vi "CSM - Request CSM to Broadcast Status Change.vi"(4 "Immediately? (F)":bool, 6 "Broadcast? (T)":bool=TRUE, 7 "Module Name":string, 8 "Error In (No Error)":errorcluster, 9 "Priority (\"Status\")":T1=enum."Status", 10 "Arguments (\"\")":string, 11 "Status":string="DoA") -> (0 "error out":errorcluster)   [LabVIEW 2017, in "Communicable State Machine.lvlib"]
doc: "Requests the CSM to send a broadcast. This VI is primarily used in CSM Multi-Loop Mode for other modules to request the CSM to issue a broadcast notifying other modules of a status change.\n\n> [!WARNING] As long as you know the module name, you can use this VI outside the CSM module to spoof a broadcast message from this module. However, this is not recommended because such logic makes the overall logic chaotic and increases debugging difficulty. Therefore, it is only recommended to use this VI in CSM Multi-Loop Mode.\n\n<b>Reference Example</b>: `4. Advance Examples\\5. Multi-Loop Module Example\\TCP Server Module(Multi-Loop Support).vi`.\n\n\n> [!NOTE] <b>CSM Multi-Loop Mode</b>\n>\n> In some scenarios, it is suitable to use multiple loops to constitute the same CSM module. For example:\n> - Retrofitting existing functional code into a CSM module. For example, TCP connection loops or DAQmx data acquisition loops. To ensure the clarity of the original logic, you can wrap the existing code in a While loop and append a CSM communication loop to implement the retrofitted functionality.\n> - In cases with high real-time requirements where a Timed Loop is needed, the CSM loop is required as a communication interface, while the Timed Loop serves as the functional loop implementation scheme.\n> - In cases where UI operations are very complex, it is recommended to separate UI operations from the CSM communication loop. The UI operation loop handles UI actions and generates inter-module messages, while the CSM loop serves as the actual functional loop.\n>\n> The Multi-Loop Support Mode API is used in such scenarios to pass internal messages between internal loops of a module or to provide CSM interface functionality for non-CSM loops.\n\n\n-- <b>Controls</b> --\n- <b>Module Name</b>: The CSM sending the status.\n- <b>Status</b>: Status to be broadcast.\n- <b>Arguments (\"\")</b>: Status arguments to be broadcast.\n- <b>Broadcast? (T)</b>: Switch input to control whether to broadcast.\n- <b>Immediately? (F)</b>: Immediate execution option. Sending immediately causes this message to be processed instantly in the CSM loop, rather than waiting for existing messages in the CSM loop to finish execution."
uses:
  Communicable State Machine.lvlib
  CSM - Broadcast Message Type.ctl
  _Support/CSMQ/_CSMOFGVOPER.ctl
  _Support/Typedef/_Cross CSM State Data.ctl
  _Support/Typedef/_CSM_MSG_TYPE.ctl
  _Support/Typedef/_Cross CSM State Response.ctl
  _Support/Typedef/_CSM_Response Source Message.ctl
  _Shared/CSM Shared.lvlib
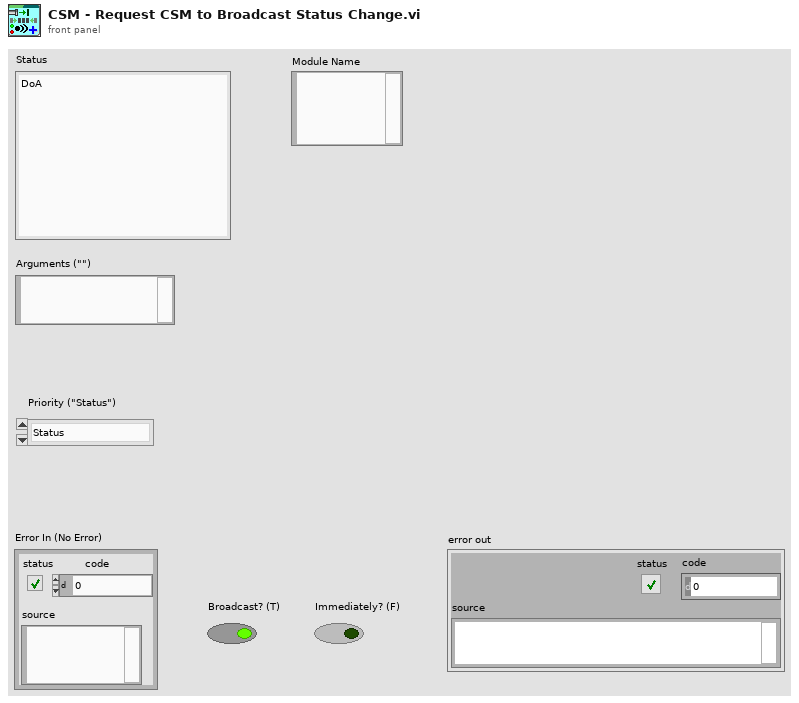
[diagram p1: front panel]
types:
  T1 = typedef "Communicable State Machine.lvlib/CSM - Broadcast Message Type.ctl" = enum16{"<Null>", "Status", "Interrupt"}
  T2 = typedef "Communicable State Machine.lvlib/_CSM_MSG_TYPE.ctl" = enum16{"Sync Message(-@)", "Async Message(->)", "Async without Response(->|)", "Async Response", "Broadcast(-><all>)", "Broadcast(-><status>)", "Broadcast(-><interrupt>)", "Append to JKISM States", "Append to JKISM States(High Priority)", "Broadcast(-><state>)"}
  T3 = typedef "Communicable State Machine.lvlib/_Cross CSM State Data.ctl" = cluster{"Msg Type":T2, "state":string, "args":string, "source":string, "RespQ":refnum<queue>, "Response For Message":T4, "Target":string}
  T4 = typedef "Communicable State Machine.lvlib/_CSM_Response Source Message.ctl" = cluster{"‘State":string, "’Arguments":string, "’Error":errorcluster}
  T5 = typedef "Communicable State Machine.lvlib/_CSMOFGVOPER.ctl" = enum16{"Create If not Exist", "Get By Name", "List", "Check If Name Exists", "Release", "Module Status", "Create Status Event Handler", "Destroy Status Event Handler", "Clear Invalid Objs"}
  T6 = typedef "Communicable State Machine.lvlib/_CSMObj.ctl" = cluster{"info":T7, "Refs":T9}
  T7 = typedef "Communicable State Machine.lvlib/_CSMObj-Info.ctl" = cluster{"Module Name":string, "Requested Name":string, "Group Name":string, "Mode":T8, "Allowed Messages":string[]}
  T8 = typedef "Communicable State Machine.lvlib/_CSM_MODE.ctl" = enum16{"Not Exist", "Stand Alone", "CSM", "Worker", "Worker Agent", "Chain Node", "Chain"}
  T9 = typedef "Communicable State Machine.lvlib/_CSMObj-Refs.ctl" = cluster{"WatchDogQ":refnum<queue>, "CSMDataDVR":refnum<data-value>, "Queue":T10, "GroupDataDVR":refnum<data-value>, "TagMap":refnum<data-value>, "ExitEvent":refnum<user-event>, "NewStateEvent":refnum<user-event>, "StatusEvent":refnum<user-event>, "InterruptEvent":refnum<user-event>}
  T10 = typedef "Communicable State Machine.lvlib/Priority Queue.ctl" = cluster{"HPriorityQ":refnum<queue>, "LowPriorityQ":refnum<queue>}
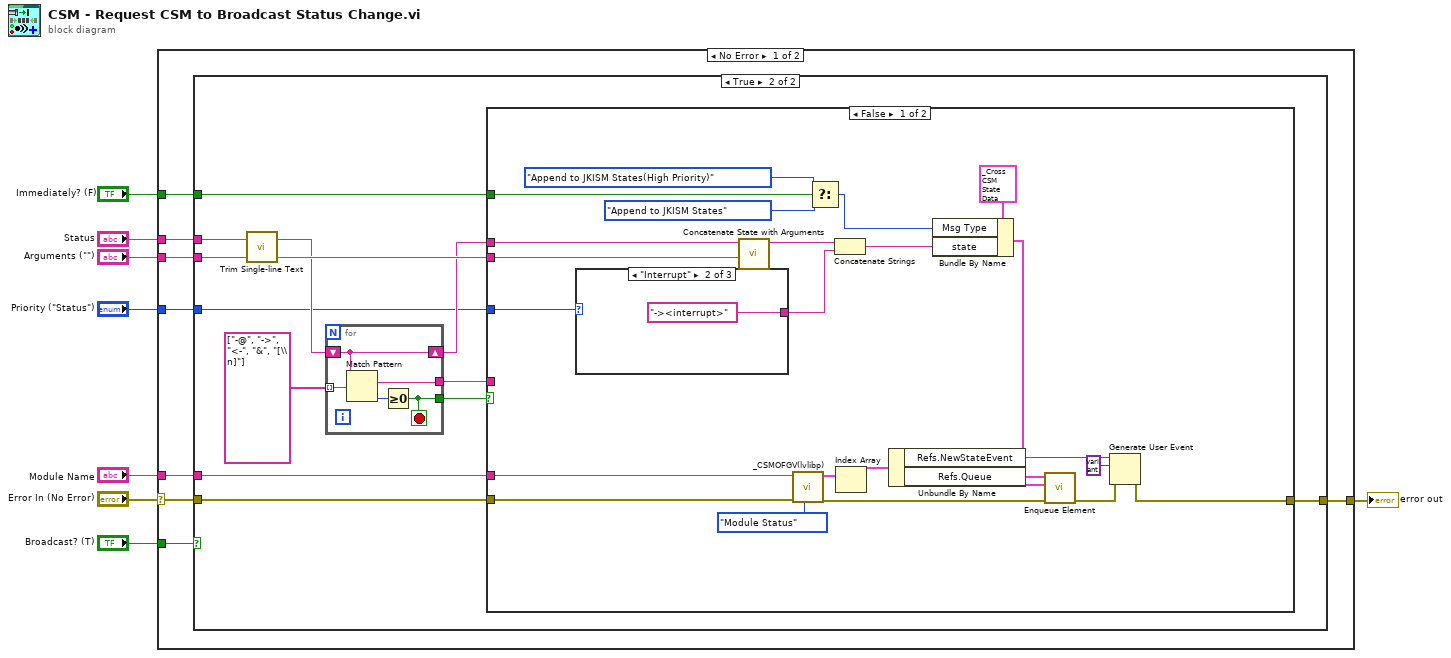
[diagram p0: block diagram]
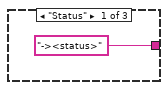
[diagram p3: hidden frame]
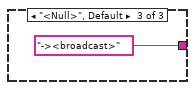
[diagram p4: hidden frame]
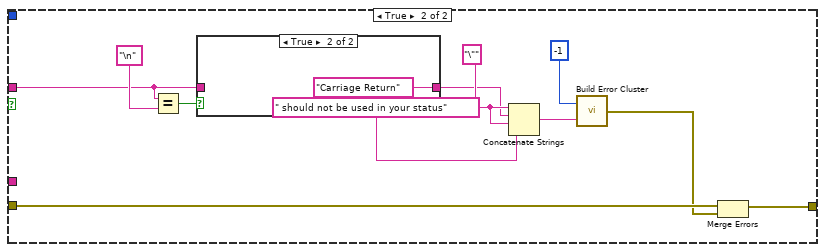
[diagram p5: hidden frame]
diagram:
  n1 = case shown="No Error" "Error In (No Error)" {
    selector: "Error In (No Error)" -> [w15 w74]
    tunnel: "Status" -> [w13 _]
    tunnel: [w16 w74] -> w6
    tunnel: "Arguments (\"\")" -> [w14 _]
    tunnel: "Module Name" -> [w12 _]
    tunnel: "Broadcast? (T)" -> [w11 _]
    tunnel: "Immediately? (F)" -> [w10 _]
    tunnel: "Priority (\"Status\")" -> [w9 _]
    frame No Error {
      n2 = case shown="True" w11 {
        tunnel: [w17 w29] -> w16
        tunnel: w15 -> [w17 w28]
        tunnel: w14 -> [_ w27]
        tunnel: w13 -> [_ w26]
        tunnel: w12 -> [_ w25]
        tunnel: w10 -> [_ w19]
        tunnel: w9 -> [_ w18]
        frame False {
        }
        frame True {
          n3 = call "Trim Single-line Text.vi"("single-line text"=w26) -> ("trimed text"=w20:string)  [unwired: 2 in]
          n4 = for {
            shift-right: [w73] -> w23
            shift-left: w20 -> [w73]
            tunnel: string[] ["-@", "->", "<-", "&", "[\\n]"] -> [w72] mode=indexing
            tunnel: [w70] -> w21
            tunnel: [w69] -> w22
            stop <- w69 stop-if-true
            n5 = Match Pattern(string=w73, regular expression=w72) -> (match substring=w70:string, offset past match=w71:i32)  [unwired: 1 in, 2 out]
            n6 = Greater Or Equal To 0?(x=w71) -> (x >= 0?=w69:bool)
          }
          n7 = case shown="False" w22 {
            tunnel: w27 -> [w32 _]
            tunnel: [w40 w58] -> w29
            tunnel: w28 -> [w45 w59]
            tunnel: w23 -> [w33 _]
            tunnel: w21 -> [_ w56]
            tunnel: w25 -> [w44 _]
            tunnel: w19 -> [w39 _]
            tunnel: w18 -> [w30 _]
            frame False {
              n8 = case shown="\"Interrupt\"" w30 {
                tunnel: ["-><status>" ("string") "-><interrupt>" ("string") "-><broadcast>" ("string")] -> w35
                frame "Status" {
                }
                frame "Interrupt" {
                }
                frame "<Null>", Default {
                }
              }
              n9 = call "Concatenate State with Arguments.vi"("Arguments"=w32, "State"=w33) -> ("State With Arguements"=w34:string)  [unwired: 9 in]
              n10 = call "_CSMOFGV(lvlibp).vi"("Operation"=_CSMOFGVOPER."Module Status", "Error In"=w45, "Name (\"\" to Use UUID) In"=w44) -> ("error out"=w46:errorcluster, "Array"=w51:T6[])  [unwired: 6 in, 1 out]
              n11 = Select(t=_CSM_MSG_TYPE."Append to JKISM States(High Priority)" ("Msg Type"), s=w39, f=_CSM_MSG_TYPE."Append to JKISM States" ("Msg Type")) -> (s? t:f=w36:T2)
              n12 = Concatenate Strings(w34, w35) -> (w31:string)
              n13 = Index Array(array=w51) -> (element=w50:T6)  [unwired: 1 in]
              n14 = Unbundle By Name(w50) -> ("Refs.NewStateEvent"=w42:refnum<user-event>, "Refs.Queue"=w49:T10)
              n15 = Bundle By Name(cluster=T3 {"Msg Type"=enum."Sync Message(-@)", "state"="", "args"="", "source"="", "RespQ"=refnum, "Response For Message"={"‘State"="", "’Arguments"="", "’Error"={"status"=FALSE, "code"=0, "source"=""}}, "Target"=""} ("element"), "Msg Type"=w36, "state"=w31) -> (w47:T3)
              n16 = call "Enqueue Element.vi"("error in (no error)"=w46, "Cross JKI State Machine State"=w47, "Priority Queue"=w49) -> ("error out"=w41:errorcluster)  [unwired: 7 in, 1 out]
              n17 = Generate User Event(user event=w42, event data cluster=variant ("event data"), error in=w41) -> (error out=w40:errorcluster)  [unwired: 1 in, 1 out]
            }
            frame True {
              w63 = "\"" ("string")
              n18 = Equal?(x=w56, y="\n" ("regular expression")) -> (x = y?=w60:bool)
              n19 = case shown="True" w60 {
                tunnel: [w67 "Carriage Return" ("State")] -> w62
                tunnel: w56 -> [w67 _]
                frame False {
                }
                frame True {
                }
              }
              n20 = Concatenate Strings(w63, w62, w63, " should not be used in your status" ("String to Prepend to source (\"\")")) -> (w64:string)
              n21 = call "Build Error Cluster.vi"("String to Prepend to Source (\"\")"=w64, "Code"=-1 ("code")) -> ("error out"=w57:errorcluster)
              n22 = Merge Errors(w59, w57) -> (w58:errorcluster)
            }
          }
        }
      }
    }
    frame Error {
    }
  }
  "error out" <- w6
